vi "MainUI.vi"() -> ()   [LabVIEW 2012]
uses:
  Status.ctl
  StimulCtrls.lvlib
  Cohort.lvclass
  Sequence.lvclass
  SubPanels/InputPadRef.vi
  UserControl/RefWorkingFile.vi
  <vilib>/Utility/miscctls.llb/LVStringsAndValuesArrayTypeDef_U8.ctl
  UserControl/LeftPanel.ctl
  CohortConfig.ctl
  UserControl/ElectdPanel.ctl
  UserControl/ElectdTerminal.ctl
  UserControl/Cohort_sm.ctl
  SEQPool/SEQPool.ctl
panel:
  out "error out":errorcluster
  out "Current Time":timestamp format="%<%X\n%x>T"
  out "Lead #":string
  out "Left Panel":T1 {"Electrode 16"."Magnitude" format="%4.2f"; "Electrode 15"."Magnitude" format="%4.2f"; "Electrode 14"."Magnitude" format="%4.2f"; "Electrode 13"."Magnitude" format="%4.2f"; "Electrode 12"."Magnitude" format="%4.2f"; "Electrode 11"."Magnitude" format="%4.2f"; "Electrode 10"."Magnitude" format="%4.2f"; "Electrode 9"."Magnitude" format="%4.2f"; "Electrode 8"."Magnitude" format="%4.2f"; "Electrode 7"."Magnitude" format="%4.2f"; "Electrode 6"."Magnitude" format="%4.2f"; "Electrode 5"."Magnitude" format="%4.2f"; "Electrode 4"."Magnitude" format="%4.2f"; "Electrode 3"."Magnitude" format="%4.2f"; "Electrode 2"."Magnitude" format="%4.2f"; "Electrode"."Magnitude" format="%4.2f"}
  out "Stimulator #":string
  out "Physician ID":string
  out "Patient ID":string
  in  "stop":bool
  out "System Status":string
  in  "Mode Tab":T4(tab)
  in  "Seqn Open":bool
  in  "SetCathode":bool
  in  "SetAnode":bool
  in  "SetHiZ":bool
  in  "Assign Ten":bool
  in  "Assign Five":bool
  in  "Assign One":bool
  in  "Electd Select None":bool
  in  "Electd Sel All":bool
  in  "Cohort Undo":bool
  in  "Seqn Check":bool
  in  "Select a Cohort to Edit":u8(ring) items=["Cohort 0"]
  in  "Cohort Clear":bool
  in  "Cohort Add":bool
  in  "Cohort Delete":bool
  in  "Sequence Operation Log Saved to":path=path "C:/Users/zhengzhang/Documents/FRI_zz/TUI Project/Data/Cohorts.txt"
  in  "Seqn New":bool
  in  "Seqn Save as":bool
  out "Sequence Waveform Preview":dbl[](graph)
  in  "Cohort Panel":T5={"Frequency [Hz]"=55.0, "Pulse Width [ms]"=450.0, "Basic Unit"={"Electrode"={"Group #"="", "T #"=0, "Magnitude"=0.0, "check"=FALSE}, "Electrode 2"={"Group #"="", "T #"=0, "Magnitude"=0.0, "check"=FALSE}, "Electrode 3"={"Group #"="", "T #"=0, "Magnitude"=0.0, "check"=FALSE}, "Electrode 4"={"Group #"="", "T #"=0, "Magnitude"=0.0, "check"=FALSE}, "Electrode 5"={"Group #"="", "T #"=0, "Magnitude"=0.0, "check"=FALSE}, "Electrode 6"={"Group #"="", "T #"=0, "Magnitude"=0.0, "check"=FALSE}, "Electrode 7"={"Group #"="", "T #"=0, "Magnitude"=0.0, "check"=FALSE}, "Electrode 8"={"Group #"="", "T #"=0, "Magnitude"=0.0, "check"=FALSE}, "Electrode 9"={"Group #"="", "T #"=0, "Magnitude"=0.0, "check"=FALSE}, "Electrode 10"={"Group #"="", "T #"=0, "Magnitude"=0.0, "check"=FALSE}, "Electrode 11"={"Group #"="", "T #"=0, "Magnitude"=0.0, "check"=FALSE}, "Electrode 12"={"Group #"="", "T #"=0, "Magnitude"=0.0, "check"=FALSE}, "Electrode 13"={"Group #"="", "T #"=0, "Magnitude"=0.0, "check"=FALSE}, "Electrode 14"={"Group #"="", "T #"=0, "Magnitude"=0.0, "check"=FALSE}, "Electrode 15"={"Group #"="", "T #"=0, "Magnitude"=0.0, "check"=FALSE}, "Electrode 16"={"Group #"="", "T #"=0, "Magnitude"=0.0, "check"=FALSE}}, "Tag"=""} {"Pulse Width [ms]" format="%#.2f"; "Basic Unit"."Electrode 16"."Magnitude" format="%4.2f"; "Basic Unit"."Electrode 15"."Magnitude" format="%4.2f"; "Basic Unit"."Electrode 14"."Magnitude" format="%4.2f"; "Basic Unit"."Electrode 13"."Magnitude" format="%4.2f"; "Basic Unit"."Electrode 12"."Magnitude" format="%4.2f"; "Basic Unit"."Electrode 11"."Magnitude" format="%4.2f"; "Basic Unit"."Electrode 10"."Magnitude" format="%4.2f"; "Basic Unit"."Electrode 9"."Magnitude" format="%4.2f"; "Basic Unit"."Electrode 8"."Magnitude" format="%4.2f"; "Basic Unit"."Electrode 7"."Magnitude" format="%4.2f"; "Basic Unit"."Electrode 6"."Magnitude" format="%4.2f"; "Basic Unit"."Electrode 5"."Magnitude" format="%4.2f"; "Basic Unit"."Electrode 4"."Magnitude" format="%4.2f"; "Basic Unit"."Electrode 3"."Magnitude" format="%4.2f"; "Basic Unit"."Electrode 2"."Magnitude" format="%4.2f"; "Basic Unit"."Electrode"."Magnitude" format="%4.2f"}
  in  "Seqn Save":bool
  in  "Sequence List":i32(listbox)
  in  "PRG Preview":bool
  in  "PRG Setting":bool
  out "Pool":T6
  in  "Remove from Program":bool
  in  "Add to Program":bool
  in  "Prog Save as":bool
  in  "Pool Edit Seqn":bool
  in  "Pool Remove":bool
  in  "Pool Add":bool
  in  "Prog New":bool
  in  "Prog Save":bool
  in  "Prog Open":bool
  in  "Cycling Mode":bool=TRUE
  in  "Emergency Stop":bool
  out "Stimulation On":bool=TRUE
  in  "Battery (%)":dbl(slide)=62.51604621309371 scale=0.0..100.0
  in  "Signal Strength":dbl(slide)=79.58921694480102 scale=0.0..100.0
  out "Elapsed Time (min.)":dbl=30.0
  out "Experiment Duration (min.)":dbl=60.0
  out "Available ASIC Unit":dbl=2.0
  out "Available Memory":string="2 MB"
  out "ASIC Unit 1 On":bool=TRUE
  out "ASIC Unit 3 On":bool
  out "ASIC Unit 5 On":bool
  out "ASIC Unit 2 On":bool=TRUE
  out "ASIC Unit 4 On":bool
  out "ASIC Unit 6 On":bool
  out "Current Protocol":string="protocol 1"
  out "Current Program":string="program 1"
  out "Current Cycle":string="cycle 3"
  # "Experiment Profile"
  # "V 0.4 (Updated 6/26/2015)"
  # "Sequence Operation"
  # "Cohort Operation"
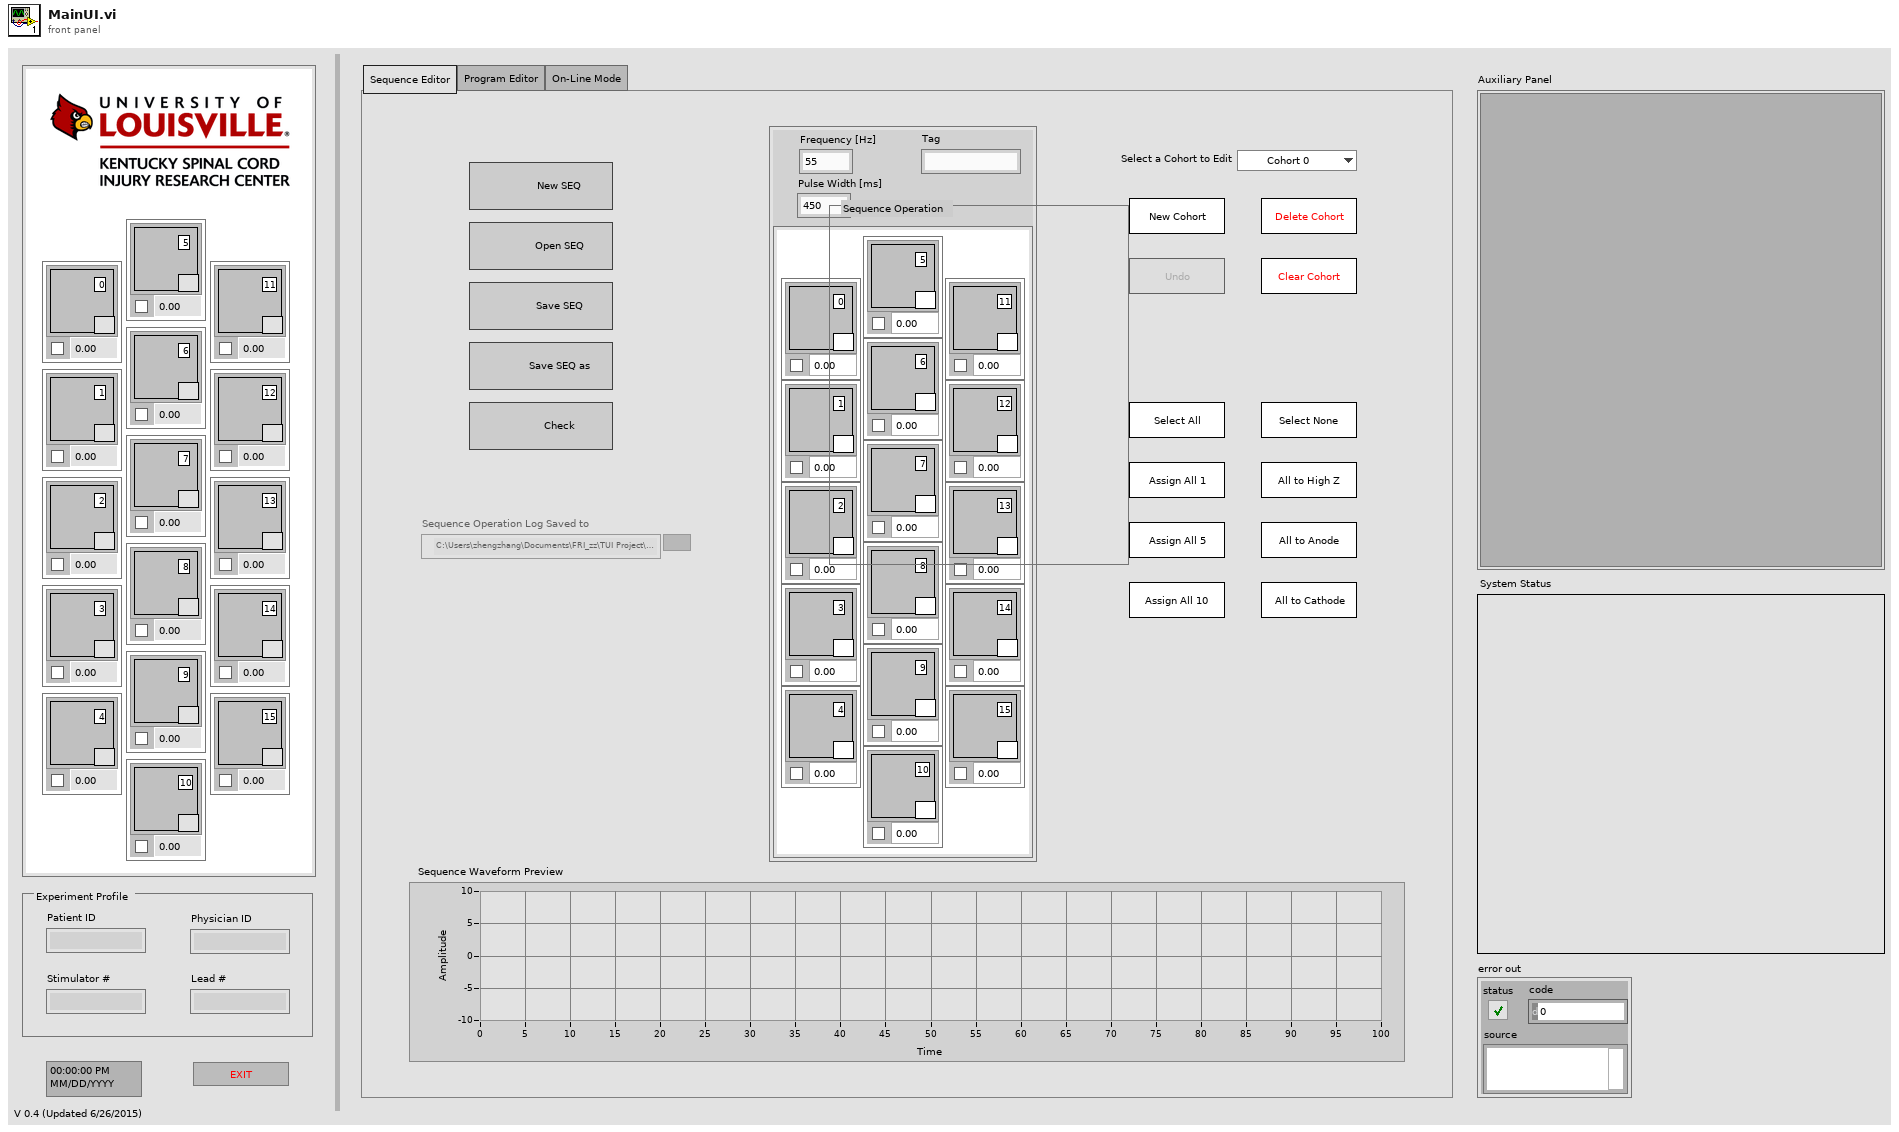
[diagram p1: front panel]
types:
  T1 = typedef "StimulCtrls.lvlib/LeftPanel.ctl" = cluster{"Electrode":T2, "Electrode 2":T2, "Electrode 3":T2, "Electrode 4":T2, "Electrode 5":T2, "Electrode 6":T2, "Electrode 7":T2, "Electrode 8":T2, "Electrode 9":T2, "Electrode 10":T2, "Electrode 11":T2, "Electrode 12":T2, "Electrode 13":T2, "Electrode 14":T2, "Electrode 15":T2, "Electrode 16":T2}
  T2 = typedef "StimulCtrls.lvlib/ElectdPanel.ctl" = cluster{"Group #":string, "T #":T3, "Magnitude":sgl, "check":bool}
  T3 = typedef "StimulCtrls.lvlib/ElectdTerminal.ctl" = u8
  T4 = enum32{"Sequence Editor", "Program Editor", "On-Line Mode"}
  T5 = typedef "StimulCtrls.lvlib/CohortConfig.ctl" = cluster{"Frequency [Hz]":sgl, "Pulse Width [ms]":sgl, "Basic Unit":T1, "Tag":string}
  T6 = typedef "StimulCtrls.lvlib/SEQPool.ctl" = cluster{"Seed 0":T7, "Seed 1":T7, "Seed 2":T7, "Seed 3":T7, "Seed 4":T7, "Seed 5":T7}
  T7 = typedef "StimulCtrls.lvlib/Cohort_sm.ctl" = cluster{"Ring 0":cluster{"T 0":T3}, "Ring 1":cluster{"T 0":T3}, "Ring 2":cluster{"T 0":T3}, "Ring 3":cluster{"T 0":T3}, "Ring 4":cluster{"T 0":T3}, "Ring 5":cluster{"T 0":T3}, "Ring 6":cluster{"T 0":T3}, "Ring 7":cluster{"T 0":T3}, "Ring 8":cluster{"T 0":T3}, "Ring 9":cluster{"T 0":T3}, "Ring 10":cluster{"T 0":T3}, "Ring 11":cluster{"T 0":T3}, "Ring 12":cluster{"T 0":T3}, "Ring 13":cluster{"T 0":T3}, "Ring 14":cluster{"T 0":T3}, "Ring 15":cluster{"T 0":T3}}
  T8 = typedef "StimulCtrls.lvlib/Status.ctl" = enum16{"SequenceOpen", "CohortShow", "Wait", "Stop", "UpdateLeftPanel", "SeqnSave", "CohortUpdate", "CohortAdd", "CohortClear", "CohortDel", "CohortBatch", "InputCall", "CohortCheck", "ProgQuit", "CohortQuickAmp", "CohortQuickState", "Initializing", "SeqnCheck", "PoolUpdate"}
  T9 = enum16{"open", "replace", "create", "open or create", "replace or create", "replace or create with confirmation"}
  T10 = enum16{"Add", "New", "Del", "Update", "Get", "Initial"}
  T11 = enum16{"Set", "Get", "Initial", "Change", "Saved"}
  T12 = enum8{"Enabled", "Disabled", "Disabled and Grayed Out"}
  T13 = typedef "LVStringsAndValuesArrayTypeDef_U8.ctl" = cluster{"String":string, "Value":u8}[]
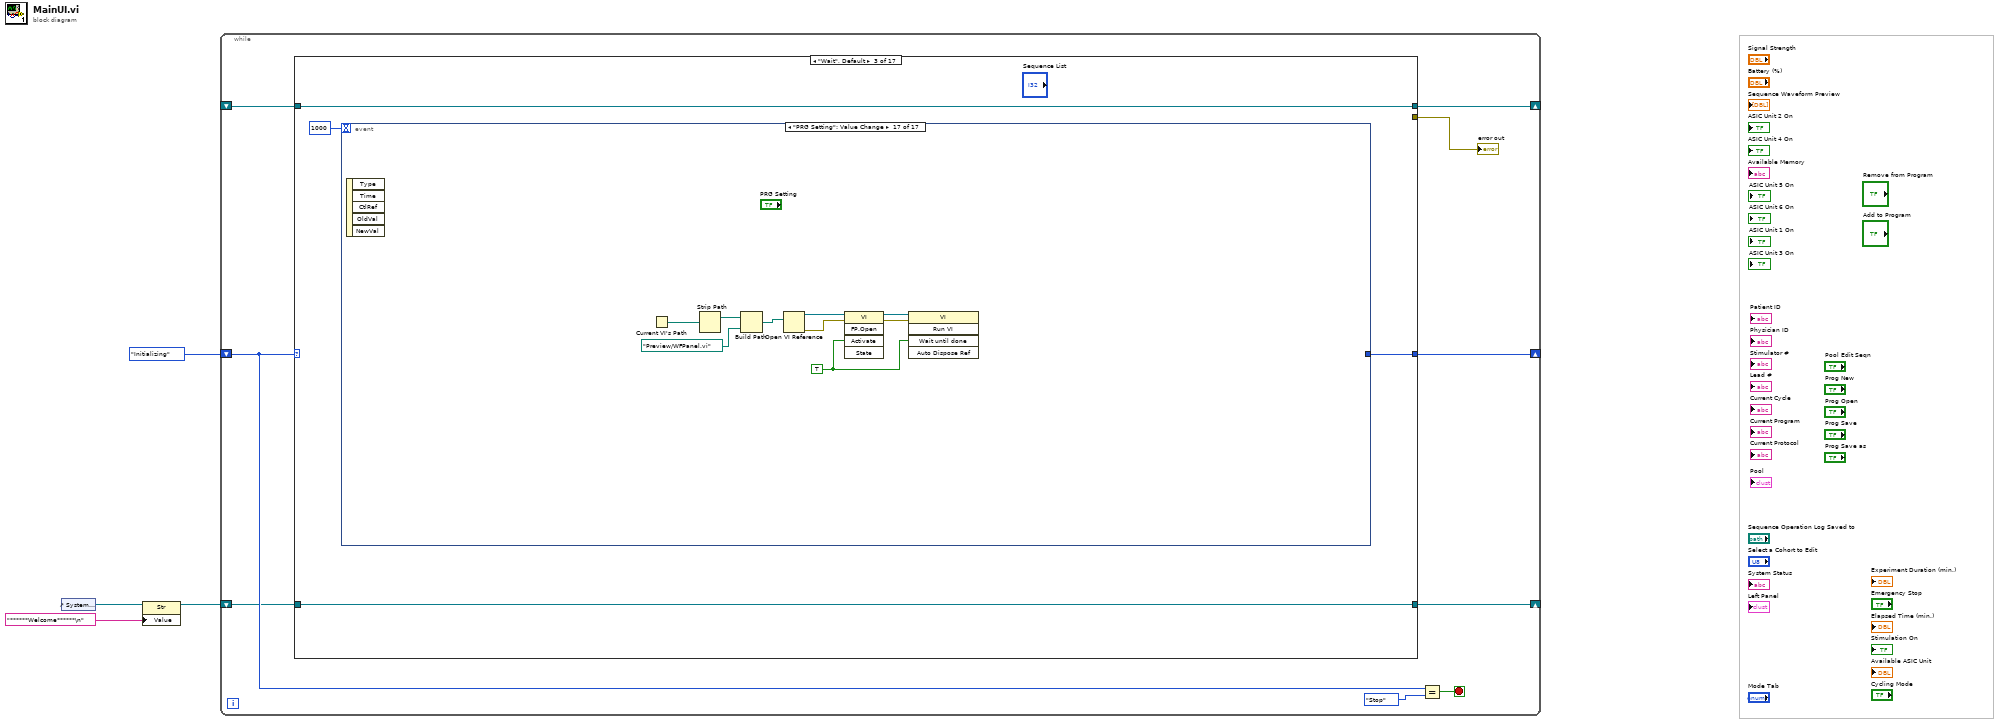
[diagram p0: block diagram]
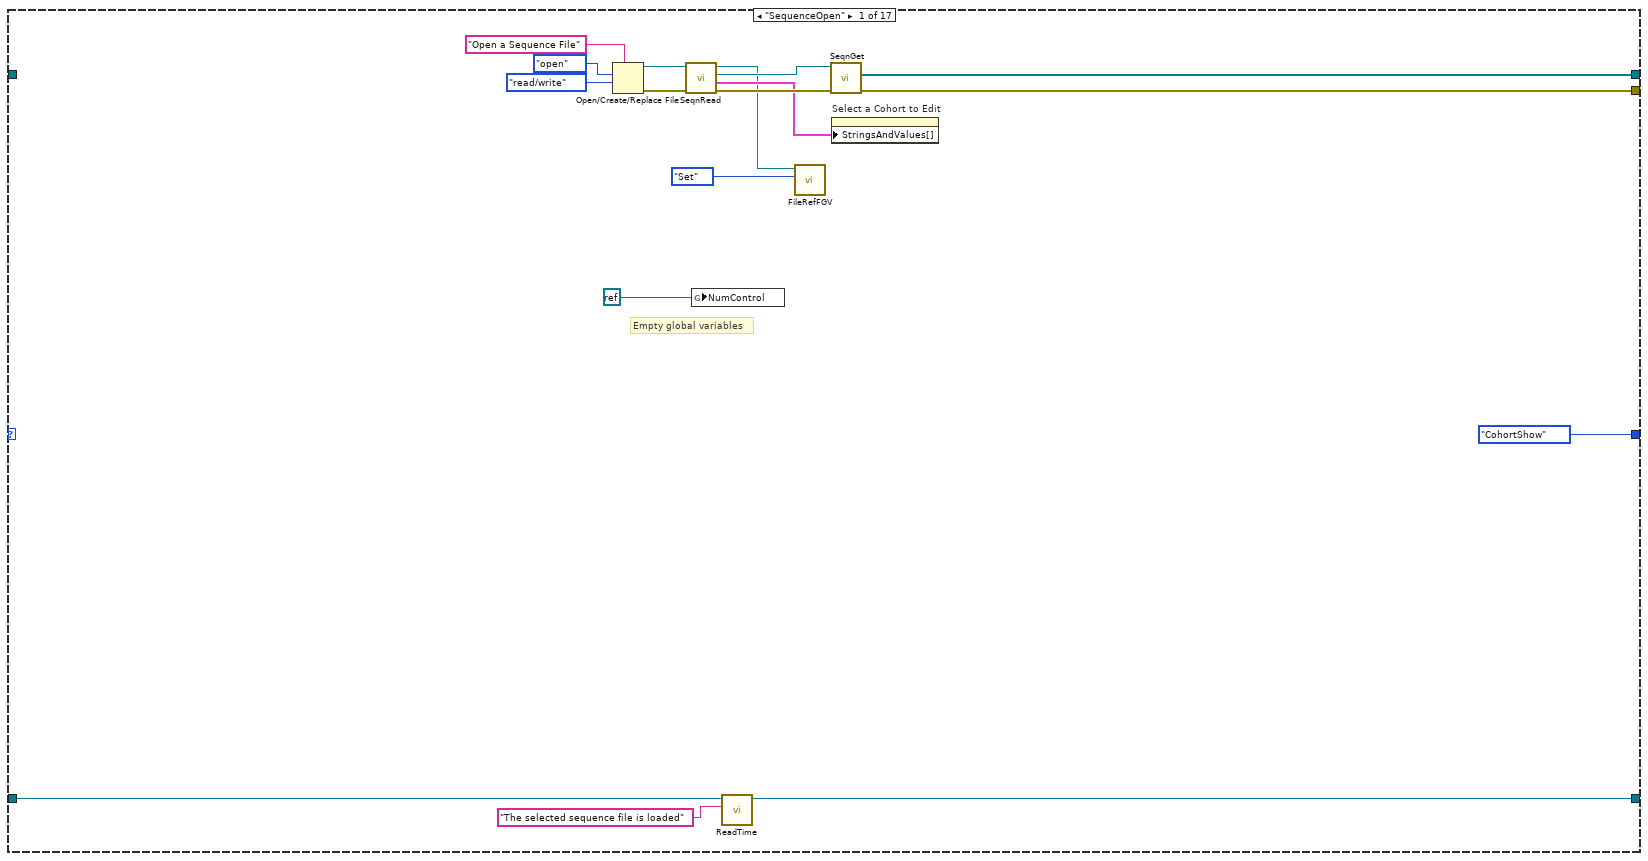
[diagram p2: hidden frame]
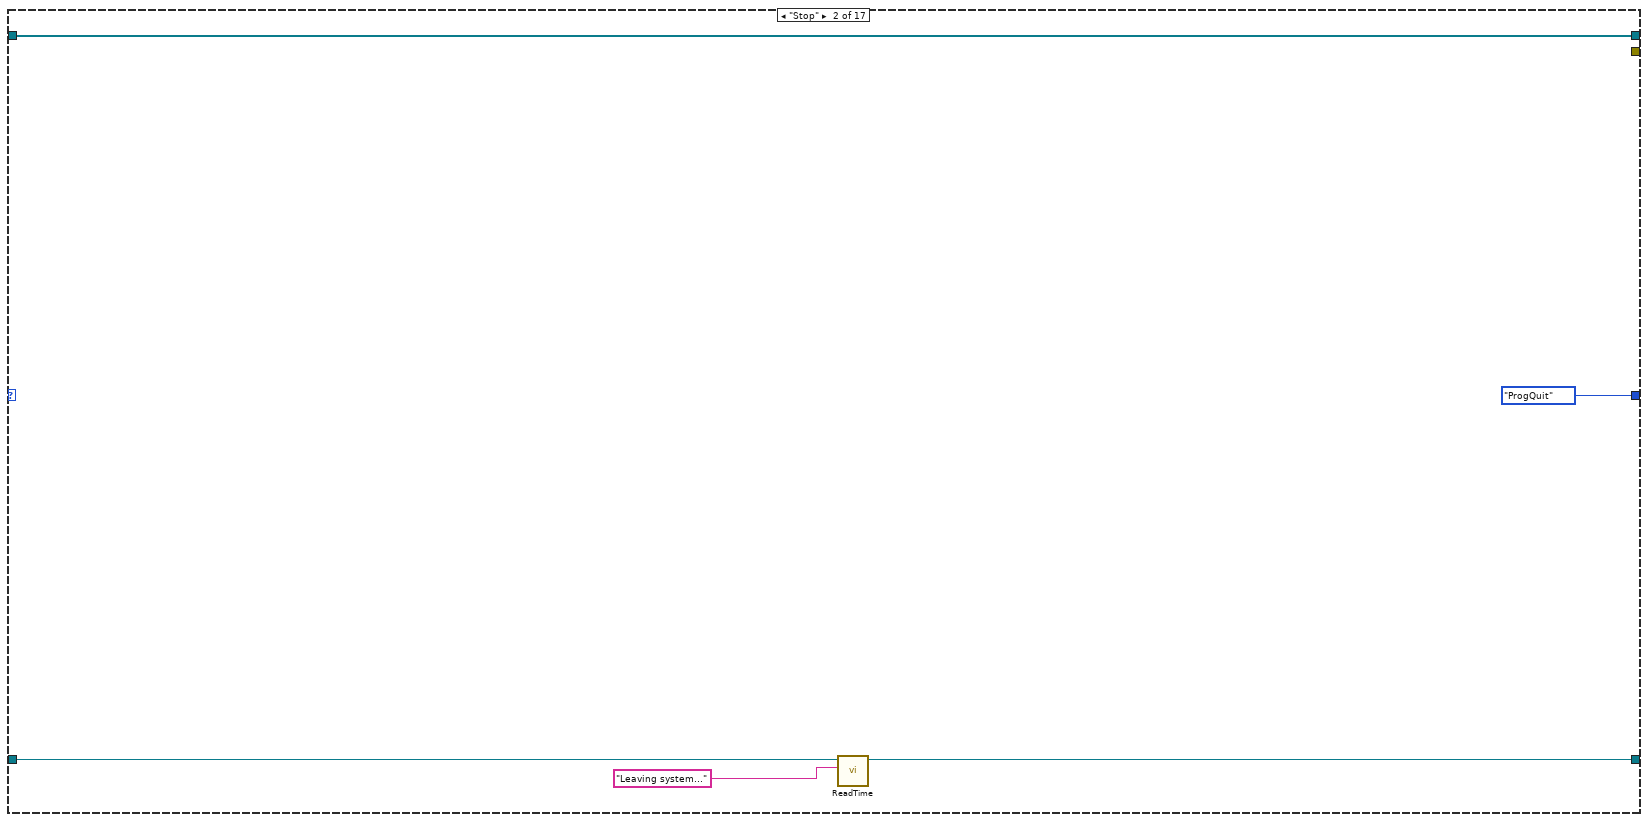
[diagram p3: hidden frame]
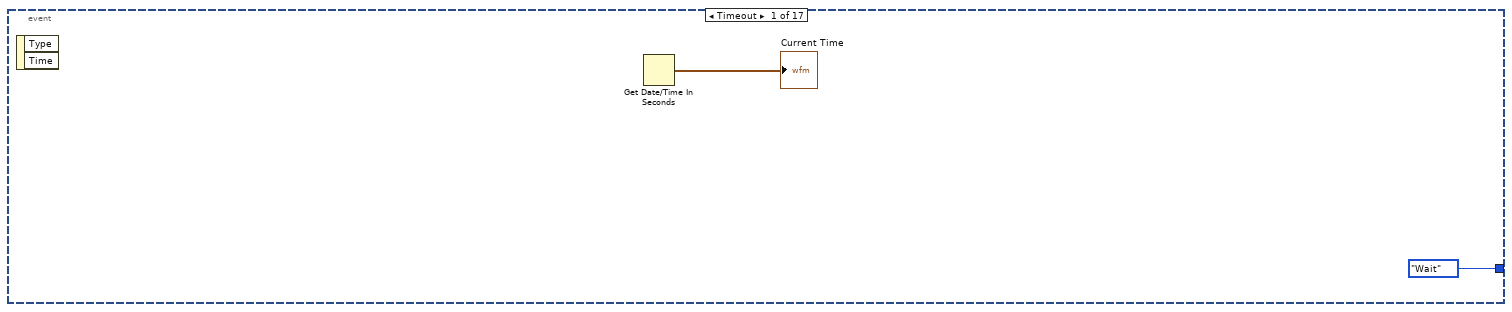
[diagram p4: hidden frame]
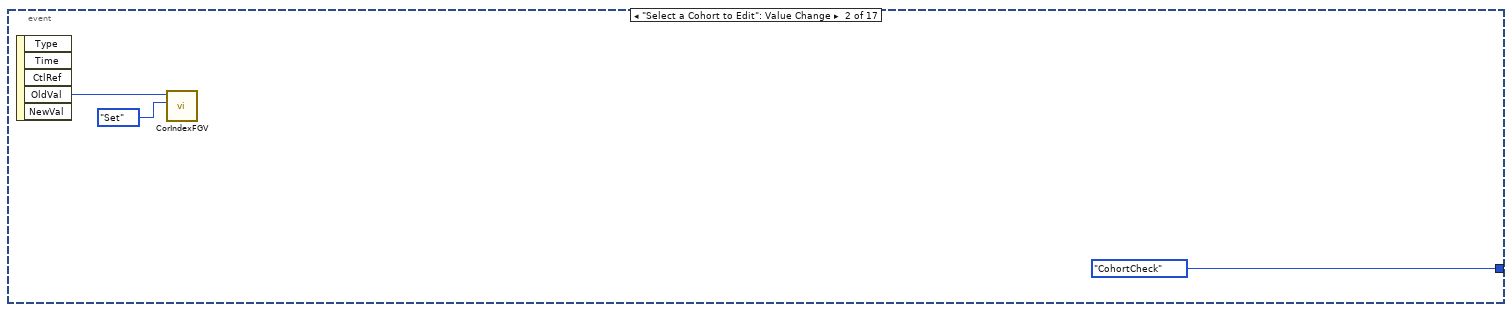
[diagram p5: hidden frame]
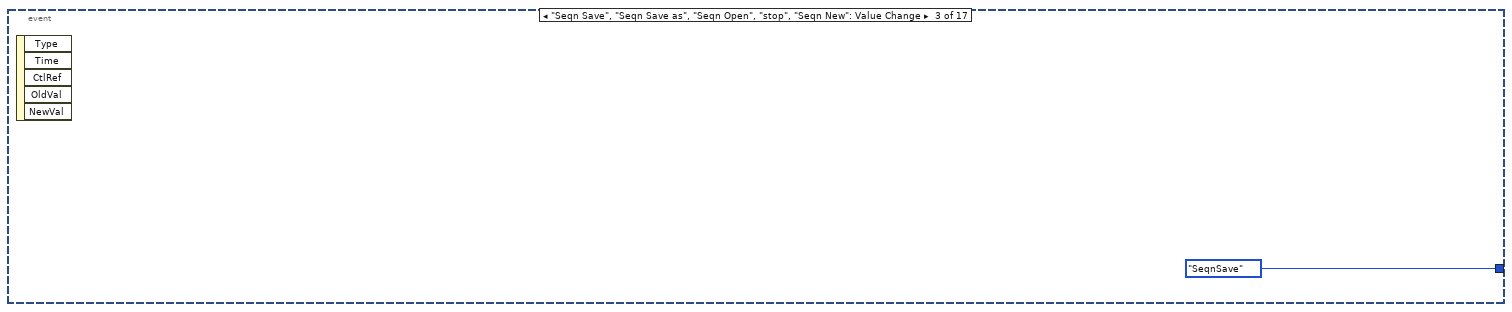
[diagram p6: hidden frame]
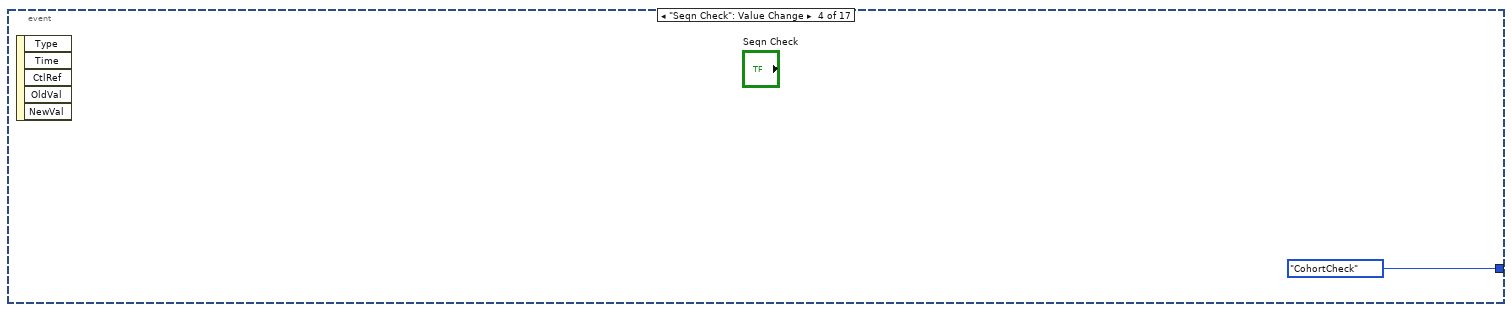
[diagram p7: hidden frame]
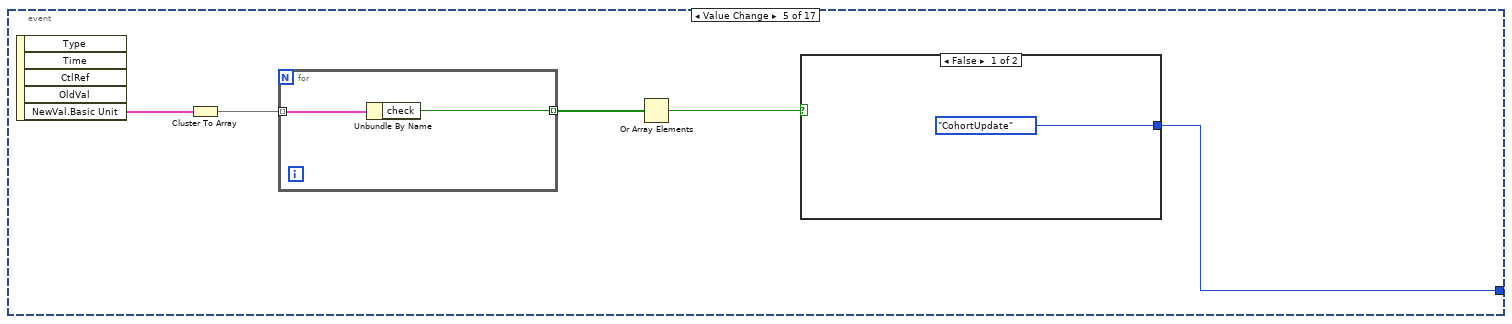
[diagram p8: hidden frame]
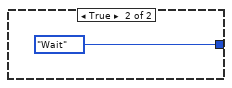
[diagram p9: hidden frame]
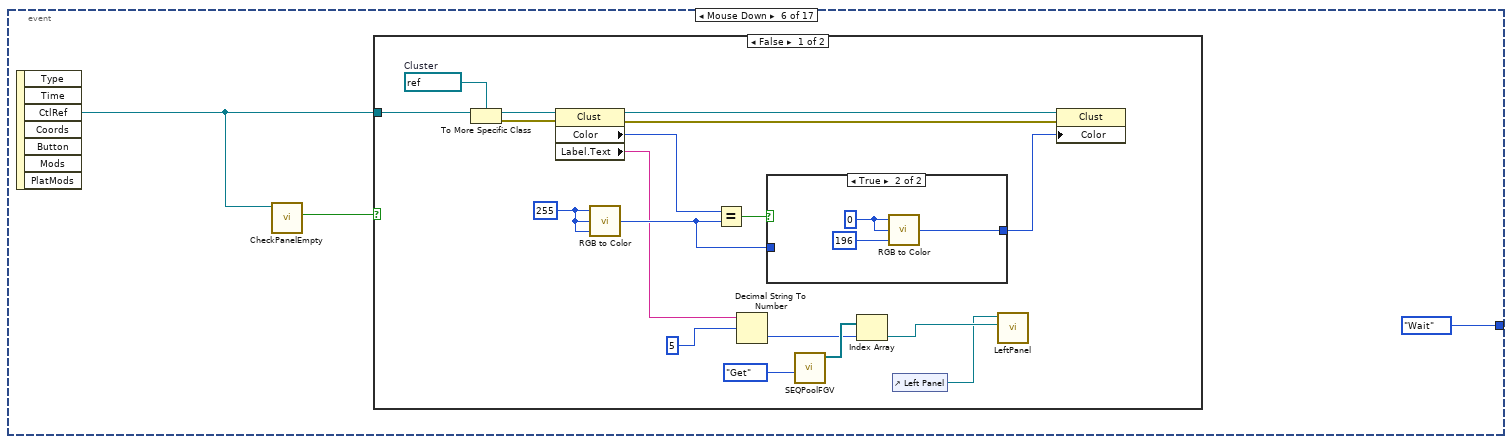
[diagram p10: hidden frame]
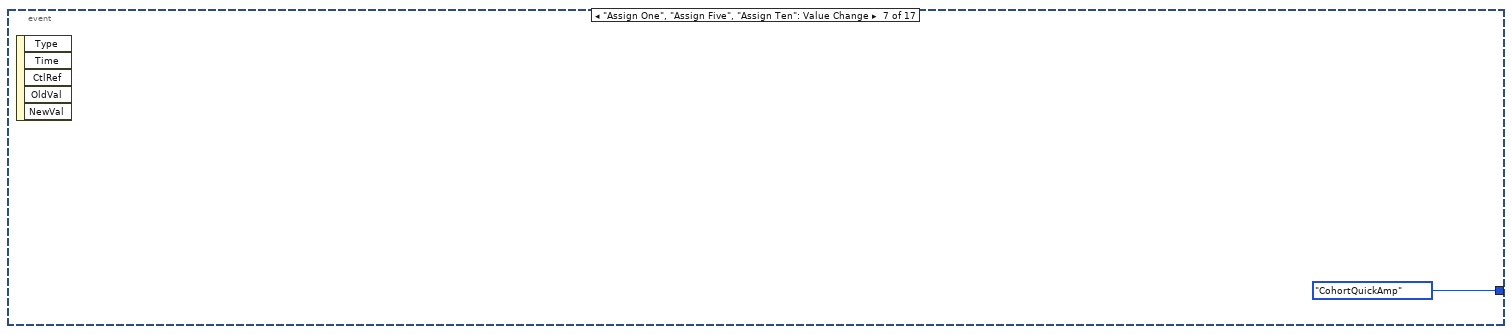
[diagram p13: hidden frame]
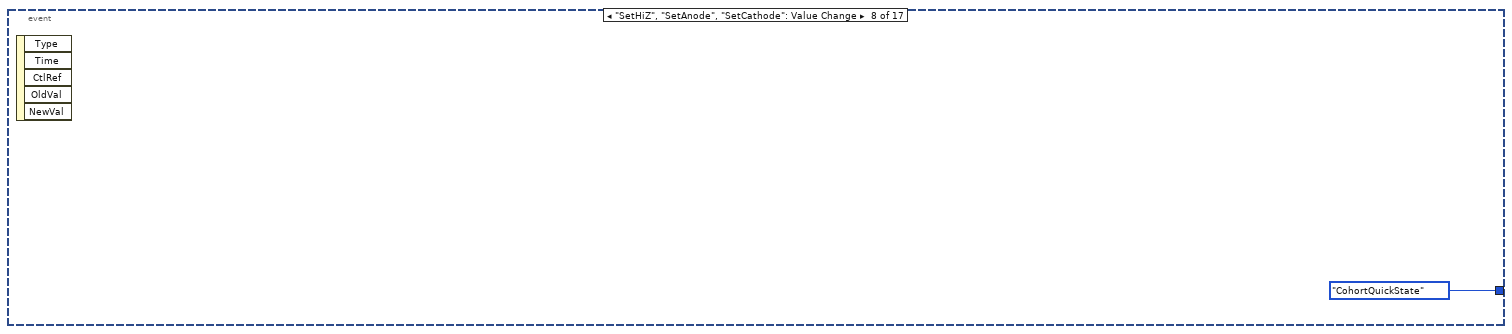
[diagram p14: hidden frame]
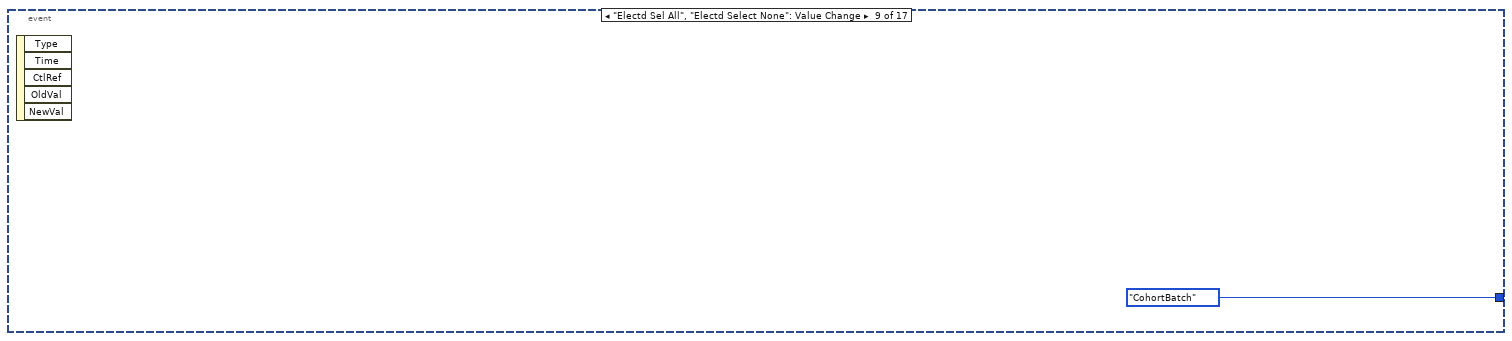
[diagram p15: hidden frame]
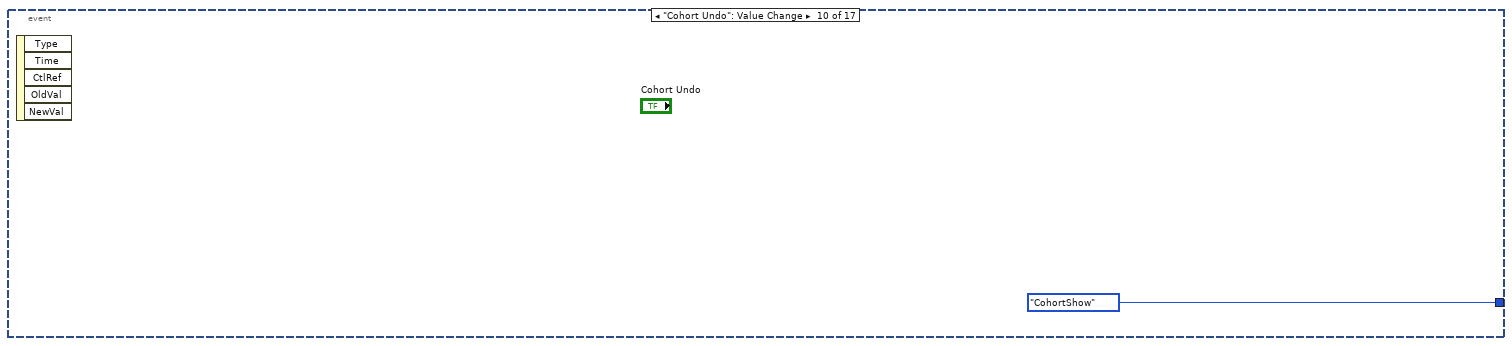
[diagram p16: hidden frame]
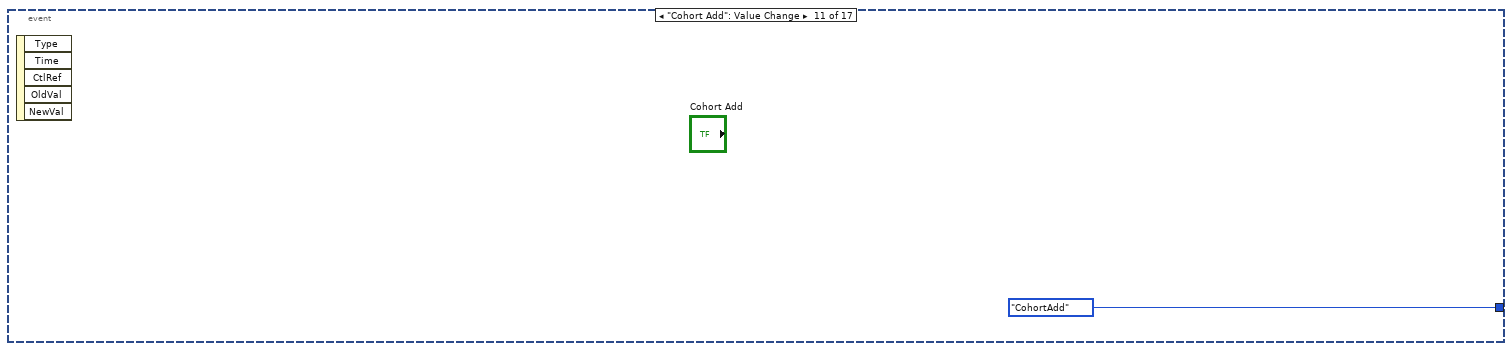
[diagram p17: hidden frame]
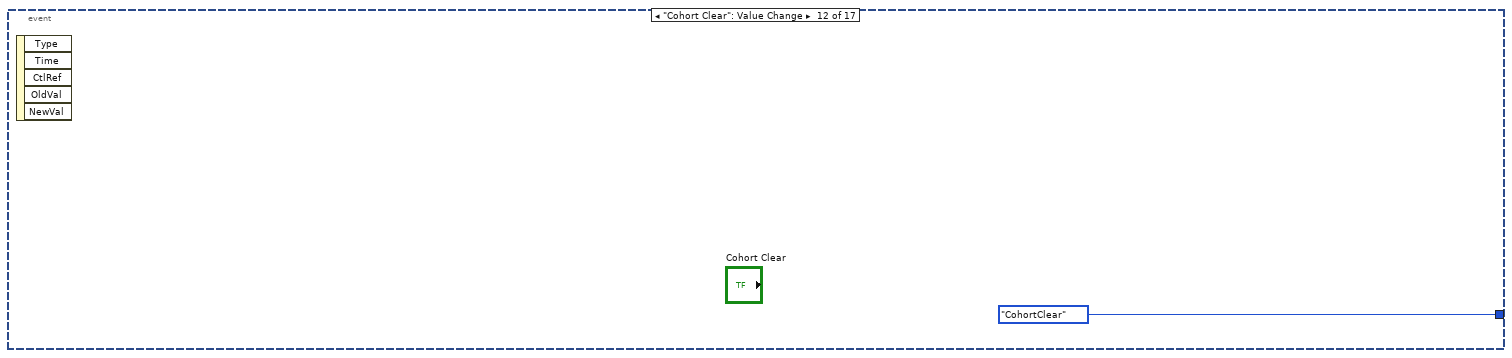
[diagram p18: hidden frame]
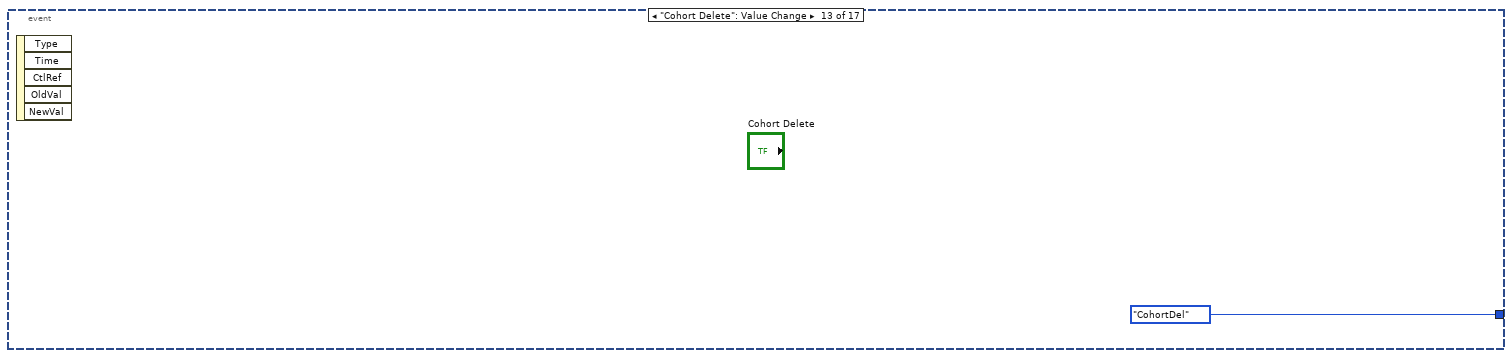
[diagram p19: hidden frame]
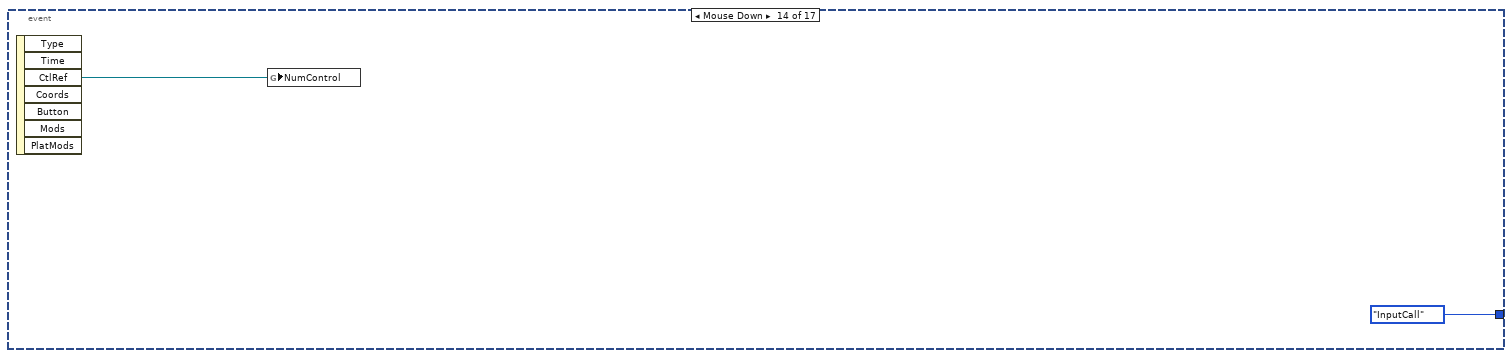
[diagram p20: hidden frame]
diagram:
  n1 = control-ref of="System Status"() -> (w1:refnum<vi>)
  n2 = property class="Str"(reference=w1, "Value"="******Welcome******\n" ("string")) -> (reference out=w3:refnum<vi>)  [unwired: 1 in, 1 out]
  n3 = while {
    shift-right: [w10] -> _
    shift-left: Status."Initializing" -> [w11]
    shift-right: [w9] -> _
    shift-left: _ -> [w8]
    shift-right: [w6] -> _
    shift-left: w3 -> [w7]
    stop <- w13 stop-if-true
    n4 = case shown="\"Wait\", Default" w11 {
      tunnel: [Status."CohortShow" Status."ProgQuit" w39 Status."Wait" w123 Status."CohortShow" Status."Wait" Status."CohortShow" Status."CohortShow" Status."UpdateLeftPanel" Status."CohortShow" Status."CohortUpdate" Status."CohortShow" Status."CohortUpdate" Status."CohortUpdate" Status."CohortShow" Status."UpdateLeftPanel"] -> w10
      tunnel: [w27 w34 w38 w114 w136 w184 w196 w233 w249 w256 w275 w307 w341 w349 w386 w418 w426] -> w9
      tunnel: w8 -> [_ w34 w38 w114 w136 w186 w196 w234 w251 w256 w276 w307 w341 w349 w386 _ w427]
      tunnel: w7 -> [w18 w32 w36 w113 w131 w174 w193 w231 w247 w254 w266 w290 w339 w348 w380 w415 w429]
      tunnel: [w17 w31 w36 w113 w130 w173 w193 w230 w246 w254 w265 w289 w339 w348 w380 w414 w429] -> w6
      tunnel: [w16 _ _ _ w122 w168 _ _ _ _ _ w281 _ _ _ _ w431] -> w5
      frame "SequenceOpen" {
        # "Empty global variables"
        n5 = Open/Create/Replace File(prompt="Open a Sequence File" ("prompt (Open existing file)"), operation (0:open)=T9."open", access (0:read/write)=enum16{"read/write", "read-only", "write-only"}."read/write") -> (refnum out=w25:refnum<file>, error out=w24:errorcluster)  [unwired: 3 in, 1 out]
        n6 = call "SeqnRead.vi"("error in (no error)"=w24, "File in Refnum"=w25) -> ("error out"=w28:errorcluster, "Cohort List"=w26:cluster{string, i32}[], "SEQ out"=w29:refnum<class "Sequence.lvclass">, "File out Refnum"=w14:refnum<file>)  [unwired: 6 in]
        n7 = global write "InputPadRef.vi" "NumControl"(refnum<k0> refnum) -> ()
        n8 = call "ReadTime.vi"("Input"="The selected sequence file is loaded", "Status in"=w18) -> ("Status out"=w17:refnum<vi>)  [unwired: 7 in]
        n9 = call "FileRefFGV.vi"("Action"=enum16{"Set", "Get", "Initial", "Change"}."Set", "File in"=w14) -> ()  [unwired: 8 in, 2 out]
        n10 = call-dynamic "SeqnGet.vi"("error in (no error)"=w28, "Sequence in"=w29) -> ("error out"=w16:errorcluster, "Cohorts"=w27:refnum<class "Cohort.lvclass">[])  [unwired: 7 in, 1 out]
        n11 = property on="Select a Cohort to Edit" class="Ring (strict)"("StringsAndValues[]"=w26) -> ()  [unwired: 2 in, 2 out]
      }
      frame "Stop" {
        n12 = call "ReadTime.vi"("Input"="Leaving system...", "Status in"=w32) -> ("Status out"=w31:refnum<vi>)  [unwired: 7 in]
      }
      frame "Wait", Default {
        n13 = event shown="[16] \"PRG Setting\": Value Change" {
          selector: _ -> [_ _ _ _ _ _ _ _ _ _ _ _ _ _ _ _ _]
          dyn-events: _ -> [_ _ _ _ _ _ _ _ _ _ _ _ _ _ _ _ _]
          timeout: 1000 -> [_ _ _ _ _ _ _ _ _ _ _ _ _ _ _ _ _]
          tunnel: [Status."Wait" Status."CohortCheck" Status."SeqnSave" Status."CohortCheck" w47 Status."Wait" Status."CohortQuickAmp" Status."CohortQuickState" Status."CohortBatch" Status."CohortShow" Status."CohortAdd" Status."CohortClear" Status."CohortDel" Status."InputCall" Status."PoolUpdate" Status."Wait" _] -> w39
          event Timeout {
            n14 = event-data() -> ()  [unwired: 1 in, 2 out]
            n15 = Get Date/Time In Seconds() -> (seconds since 1Jan1904=→"Current Time":timestamp)
          }
          event "Select a Cohort to Edit": Value Change {
            n16 = event-data() -> ("OldVal"=w43:u8)  [unwired: 1 in, 4 out]
            n17 = call "CorIndexFGV.vi"("Action"=enum16{"Set", "Get"}."Set", "Cohort Index"=w43) -> ()  [unwired: 9 in, 1 out]
          }
          event "Seqn Save", "Seqn Save as", "Seqn Open", "stop", "Seqn New": Value Change {
            n18 = event-data() -> ()  [unwired: 1 in, 5 out]
          }
          event "Seqn Check": Value Change {
            n19 = event-data() -> ()  [unwired: 1 in, 5 out]
          }
          event Value Change {
            n20 = event-data() -> ("NewVal.Basic Unit"=w51:T1)  [unwired: 1 in, 4 out]
            n21 = Cluster To Array(cluster=w51) -> (array=w50:T2[])
            n22 = for {
              tunnel: w50 -> [w55] mode=indexing
              tunnel: [w54] -> w49 mode=indexing
              n23 = Unbundle By Name(w55) -> ("check"=w54:bool)
            }
            n24 = Or Array Elements(Boolean array=w49) -> (logical OR=w48:bool)
            n25 = case shown="False" w48 {
              tunnel: [Status."CohortUpdate" Status."Wait"] -> w47
              frame False {
              }
              frame True {
              }
            }
          }
          event Mouse Down {
            n26 = event-data() -> ("CtlRef"=w57:refnum<vi>)  [unwired: 1 in, 6 out]
            n27 = call "CheckPanelEmpty.vi"("Panel in"=w57) -> ("Empty?"=w56:bool)  [unwired: 10 in]
            n28 = case shown="False" w56 {
              tunnel: w57 -> [w66 _]
              frame False {
                w73 = u8 255 ("R")
                w74 = refnum<vi> refnum  # Cluster
                n29 = To More Specific Class(target class=w74, reference=w66) -> (specific class reference=w76:refnum<vi>, error out=w75:errorcluster)  [unwired: 1 in]
                n30 = property class="Clust"(reference=w76, error in=w75) -> (reference out=w70:refnum<vi>, error out=w69:errorcluster, "Color"=w72:u32, "Label.Text"=w60:string)
                n31 = call <vilib>:"RGB to Color.vi"("B"=w73, "G"=w73, "R"=w73) -> ("Color"=w68:u32)
                n32 = Equal?(x=w72, y=w68) -> (x = y?=w71:bool)
                n33 = Decimal String To Number(string=w60, offset=5 ("offset (0)")) -> (number=w63:i32)  [unwired: 1 in, 1 out]
                n34 = case shown="True" w71 {
                  tunnel: w68 -> [w77 _]
                  tunnel: [w77 w78] -> w67
                  frame False {
                  }
                  frame True {
                    w80 = u8 0 ("R")
                    n35 = call <vilib>:"RGB to Color.vi"("B"=u8 196, "G"=w80, "R"=w80) -> ("Color"=w78:u32)
                  }
                }
                n36 = call "SEQPoolFGV.vi"("Action"=T10."Get") -> ("SEQ out"=w64:refnum<class "Sequence.lvclass">[])  [unwired: 10 in]
                n37 = Index Array(array=w64, index=w63) -> (element=w62:refnum<class "Sequence.lvclass">)
                n38 = control-ref of="Left Panel"() -> (w61:refnum<vi>)
                n39 = call "LeftPanel.vi"("Seqn in"=w62, "LP Refnum"=w61) -> ()  [unwired: 10 in]
                n40 = property class="Clust"(reference=w70, error in=w69, "Color"=w67) -> ()  [unwired: 2 out]
              }
              frame True {
              }
            }
          }
          event "Assign One", "Assign Five", "Assign Ten": Value Change {
            n41 = event-data() -> ()  [unwired: 1 in, 5 out]
          }
          event "SetHiZ", "SetAnode", "SetCathode": Value Change {
            n42 = event-data() -> ()  [unwired: 1 in, 5 out]
          }
          event "Electd Sel All", "Electd Select None": Value Change {
            n43 = event-data() -> ()  [unwired: 1 in, 5 out]
          }
          event "Cohort Undo": Value Change {
            n44 = event-data() -> ()  [unwired: 1 in, 5 out]
          }
          event "Cohort Add": Value Change {
            n45 = event-data() -> ()  [unwired: 1 in, 5 out]
          }
          event "Cohort Clear": Value Change {
            n46 = event-data() -> ()  [unwired: 1 in, 5 out]
          }
          event "Cohort Delete": Value Change {
            n47 = event-data() -> ()  [unwired: 1 in, 5 out]
          }
          event Mouse Down {
            n48 = event-data() -> ("CtlRef"=w88:refnum<vi>)  [unwired: 1 in, 6 out]
            n49 = global write "InputPadRef.vi" "NumControl"(w88) -> ()
          }
          event "Pool Add", "Pool Remove": Value Change {
            n50 = event-data() -> ()  [unwired: 1 in, 5 out]
          }
          event "PRG Preview": Value Change {
            n51 = event-data() -> ()  [unwired: 1 in, 5 out]
            n52 = Current VI's Path() -> (path=w99:path)
            n53 = Strip Path(path=w99) -> (stripped path=w100:path)  [unwired: 1 out]
            n54 = Build Path(base path=w100, name or relative path=path "Preview/WFPanel.vi" ("vi path")) -> (appended path=w98:path)
            n55 = Open VI Reference(vi path=w98) -> (vi reference=w96:refnum<vi>, error out=w95:errorcluster)  [unwired: 5 in]
            n56 = invoke class="VI" method="FP.Open"(reference=w96, error in=w95, "Activate"=TRUE ("Wait Until Done")) -> (reference out=w93:refnum<vi>, error out=w92:errorcluster)  [unwired: 2 in, 3 out]
            n57 = invoke class="VI" method="Run VI"(reference=w93, error in=w92, "Wait until done"=FALSE ("Wait Until Done")) -> ()  [unwired: 2 in, 5 out]
          }
          event "PRG Setting": Value Change {
            w102 = TRUE ("Wait Until Done")
            n58 = event-data() -> ()  [unwired: 1 in, 5 out]
            n59 = Current VI's Path() -> (path=w108:path)
            n60 = Strip Path(path=w108) -> (stripped path=w109:path)  [unwired: 1 out]
            n61 = Build Path(base path=w109, name or relative path=path "Preview/WFPanel.vi" ("vi path")) -> (appended path=w107:path)
            n62 = Open VI Reference(vi path=w107) -> (vi reference=w106:refnum<vi>, error out=w105:errorcluster)  [unwired: 5 in]
            n63 = invoke class="VI" method="FP.Open"(reference=w106, error in=w105, "Activate"=w102) -> (reference out=w104:refnum<vi>, error out=w103:errorcluster)  [unwired: 2 in, 3 out]
            n64 = invoke class="VI" method="Run VI"(reference=w104, error in=w103, "Wait until done"=w102) -> ()  [unwired: 2 in, 5 out]
          }
        }
      }
      frame "UpdateLeftPanel" {
        n65 = call "SeqnSet.vi"("Sequence"=w114) -> ("Sequence out"=w112:refnum<class "Sequence.lvclass">)  [unwired: 8 in, 1 out]
        n66 = control-ref of="Left Panel"() -> (w111:refnum<vi>)
        n67 = call "LeftPanel.vi"("Seqn in"=w112, "LP Refnum"=w111) -> ()  [unwired: 10 in]
      }
      frame "SeqnSave" {
        # "Save file?"
        # "File changed?"
        n68 = call "FileRefFGV.vi"("Action"=enum16{"Set", "Get", "Initial", "Change"}."Get") -> ("Changed?"=w120:bool)  [unwired: 9 in, 1 out]
        n69 = case shown="True" w120 {
          tunnel: [FALSE ("T button?") w140] -> w117
          frame False {
          }
          frame True {
            n70 = Two Button Dialog(message="Save current edit?", 1:"No" ("F button name (\"Cancel\")"), 2:"Yes" ("F button name (\"Cancel\")")) -> (T button?=w140:bool)
          }
        }
        n71 = Compound Arithmetic op=OR("Seqn Save as", w117, "Seqn Save") -> (w119:bool)
        n72 = case shown="True" w119 {
          tunnel: w136 -> [_ w150]
          tunnel: "Seqn Save as" -> [_ w148]
          tunnel: [errorcluster {"status"=FALSE, "code"=0, "source"=""} ("error out") w144] -> w122
          frame False {
          }
          frame True {
            n73 = case shown="False" w148 {
              tunnel: [w152 w158] -> w149
              tunnel: [w151 w157] -> w147
              frame True {
                n74 = Open/Create/Replace File(prompt="Create a New Cohort File", operation (0:open)=T9."replace or create") -> (refnum out=w152:refnum<file>, error out=w151:errorcluster)  [unwired: 4 in, 1 out]
                n75 = global write "RefWorkingFile.vi" "Working File Refnum"(w152) -> ()
              }
              frame False {
                n76 = call "FileRefFGV.vi"("Action"=enum16{"Set", "Get", "Initial", "Change"}."Get") -> ("File out"=w155:refnum<file>)  [unwired: 9 in, 1 out]
                n77 = Not Equal?(x=w155, y=refnum<k0> refnum) -> (x != y?=w159:bool)
                n78 = case shown="False" w159 {
                  tunnel: w155 -> [_ w166]
                  tunnel: [w162 w166] -> w158
                  tunnel: [w161 errorcluster {"status"=FALSE, "code"=0, "source"=""} ("error constant")] -> w157
                  frame False {
                    # "If file is no opened"
                    n79 = Open/Create/Replace File(prompt="Create a New Cohort File", operation (0:open)=T9."replace or create") -> (refnum out=w162:refnum<file>, error out=w161:errorcluster)  [unwired: 4 in, 1 out]
                    n80 = global write "RefWorkingFile.vi" "Working File Refnum"(w162) -> ()
                  }
                  frame True {
                  }
                }
              }
            }
            n81 = call "SeqnSet.vi"("Sequence"=w150, "error in (no error)"=w147) -> ("Sequence out"=w146:refnum<class "Sequence.lvclass">, "error out"=w145:errorcluster)  [unwired: 7 in]
            n82 = call "SeqnWrite.vi"("error in (no error)"=w145, "Seqn in"=w146, "File in Refnum"=w149) -> ("error out"=w144:errorcluster)  [unwired: 8 in]
            n83 = call "FileRefFGV.vi"("Action"=T11."Saved") -> ()  [unwired: 9 in, 2 out]
          }
        }
        n84 = call "ReadTime.vi"("Input"="The current sequence is saved", "Status in"=w131) -> ("Status out"=w130:refnum<vi>)  [unwired: 7 in]
        n85 = Select(t=Status."Initializing", s="Seqn New", f=Status."Wait") -> (s? t:f=w128:T8)
        n86 = Select(t=Status."SequenceOpen", s="Seqn Open", f=w128) -> (s? t:f=w126:T8)
        n87 = Select(t=Status."Stop", s="stop", f=w126) -> (s? t:f=w123:T8)
      }
      frame "CohortAdd" {
        w188 = u8 1 ("Set Pulse Frequency")
        # "To create an automatic tag for the new cohort in the ring\nNew cohort will be appended to the sequence"
        # "Append the new cohort to the array"
        # "Initialize a new, empty cohort"
        n88 = control-ref of="Select a Cohort to Edit"() -> (w183:refnum<vi>)
        n89 = property class="Ring (strict)"(reference=w183) -> (reference out=w182:refnum<vi>, error out=w169:errorcluster, "StringsAndValues[]"=w177:T13, "NumItems"=w172:u32)  [unwired: 1 in]
        n90 = Initialize Array(-1, 16 ("dimension size")) -> (w189:i32[])
        n91 = Number To Decimal String(number=w172, width (-)=i16 2) -> (decimal integer string=w179:string)
        n92 = Concatenate Strings("Cohort", w179) -> (w170:string)
        n93 = call "CohortSet.vi"("Set COR Tag"=w170, "Set Electrodes"=w189, "Set Pulse Width"=w188, "Set Pulse Frequency"=w188) -> ("Cohort out"=w185:refnum<class "Cohort.lvclass">)  [unwired: 6 in, 1 out]
        n94 = Bundle(w170, "NumItems"=w172) -> (w176:cluster{string, "NumItems":u32})  [unwired: 1 in]
        n95 = call "CorIndexFGV.vi"("Action"=enum16{"Set", "Get"}."Set", "Cohort Index"=w172) -> ()  [unwired: 9 in, 1 out]
        n96 = call "FileRefFGV.vi"("Action"=enum16{"Set", "Get", "Initial", "Change"}."Change") -> ()  [unwired: 9 in, 2 out]
        n97 = Build Array (concatenate)(w177, w176) -> (w178:cluster{"String":string, "NumItems":u32}[])
        n98 = call "ReadTime.vi"("Input"="A empty cohort is appended to the current sequence", "Status in"=w174) -> ("Status out"=w173:refnum<vi>)  [unwired: 7 in]
        n99 = Insert Into Array(array=w186, new element=w185) -> (w184:refnum<class "Cohort.lvclass">[])  [unwired: 1 in]
        n100 = property class="Ring (strict)"(reference=w182, error in=w169, "StringsAndValues[]"=w178) -> (error out=w168:errorcluster)  [unwired: 1 out]
      }
      frame "CohortBatch" {
        w199 = refnum<vi> refnum  # Cluster
        # "Electrode"
        n101 = control-ref of="Cohort Panel"() -> (w204:refnum<vi>)
        n102 = property class="Clust (strict)"(reference=w204) -> ("Controls[]"=w203:refnum<vi>[])  [unwired: 1 in, 2 out]
        n103 = Index Array(array=w203, index=2) -> (element=w201:refnum<vi>)
        n104 = To More Specific Class(target class=w199, reference=w201) -> (specific class reference=w200:refnum<vi>)  [unwired: 1 in, 1 out]
        n105 = property class="Clust"(reference=w200) -> ("Controls[]"=w198:refnum<vi>[])  [unwired: 1 in, 2 out]
        n106 = for {
          tunnel: w198 -> [w220] mode=indexing
          tunnel: "Electd Sel All" -> [w209]
          tunnel: "Electd Select None" -> [w205]
          w216 = refnum<vi> refnum  # Boolean
          w221 = refnum<vi> refnum  # Cluster
          # "Select All"
          # "Select None"
          # "Checkbox"
          n107 = To More Specific Class(target class=w221, reference=w220) -> (specific class reference=w219:refnum<vi>)  [unwired: 1 in, 1 out]
          n108 = property class="Clust"(reference=w219) -> ("Controls[]"=w217:refnum<vi>[])  [unwired: 1 in, 2 out]
          n109 = Index Array(array=w217, index=3) -> (element=w215:refnum<vi>)
          n110 = To More Specific Class(target class=w216, reference=w215) -> (specific class reference=w206:refnum<vi>)  [unwired: 1 in, 1 out]
          n111 = case shown="True" w205 {
            tunnel: w206 -> [_ w223]
            frame False {
            }
            frame True {
              n112 = property class="Bool"(reference=w223, "Value"=FALSE) -> ()  [unwired: 1 in, 2 out]
            }
          }
          n113 = property class="Bool"(reference=w206) -> (reference out=w208:refnum<vi>, "DisabledEnum"=w214:T12)  [unwired: 1 in, 1 out]
          n114 = Equal?(x=w214, y=T12."Enabled") -> (x = y?=w212:bool)
          n115 = Select(t=TRUE, s=w212, f=FALSE) -> (s? t:f=w207:bool)
          n116 = case shown="True" w209 {
            tunnel: w208 -> [_ w225]
            tunnel: w207 -> [_ w224]
            frame False {
            }
            frame True {
              n117 = property class="Bool"(reference=w225, "Value"=w224) -> ()  [unwired: 1 in, 2 out]
            }
          }
        }
        n118 = call "FileRefFGV.vi"("Action"=enum16{"Set", "Get", "Initial", "Change"}."Change") -> ()  [unwired: 9 in, 2 out]
      }
      frame "CohortClear" {
        w236 = u8 1 ("Set Pulse Frequency")
        n119 = Initialize Array(-1, 16 ("dimension size")) -> (w237:i32[])
        n120 = call "CohortSet.vi"("Set COR Tag"="", "Set Electrodes"=w237, "Set Pulse Width"=w236, "Set Pulse Frequency"=w236) -> ("Cohort out"=w235:refnum<class "Cohort.lvclass">)  [unwired: 6 in, 1 out]
        n121 = call "CorIndexFGV.vi"("Action"=enum16{"Set", "Get"}."Get") -> ("New Index"=w229:u8)  [unwired: 10 in]
        n122 = call "ReadTime.vi"("Input"="The current cohort is cleared", "Status in"=w231) -> ("Status out"=w230:refnum<vi>)  [unwired: 7 in]
        n123 = call "FileRefFGV.vi"("Action"=enum16{"Set", "Get", "Initial", "Change"}."Change") -> ()  [unwired: 9 in, 2 out]
        n124 = Replace Array Subset(array=w234, new element=w235, index=w229) -> (w233:refnum<class "Cohort.lvclass">[])
      }
      frame "CohortDel" {
        n125 = property on="Select a Cohort to Edit" class="Ring (strict)"() -> ("Strings []"=w244:string[])  [unwired: 2 in, 2 out]
        n126 = call "CorIndexFGV.vi"("Action"=enum16{"Set", "Get", "Del"}."Del") -> ("New Index"=w243:u8)  [unwired: 10 in]
        n127 = call "FileRefFGV.vi"("Action"=enum16{"Set", "Get", "Initial", "Change"}."Change") -> ()  [unwired: 9 in, 2 out]
        n128 = Delete From Array(array=w251, index=w243) -> (array with subset deleted=w249:refnum<class "Cohort.lvclass">[])  [unwired: 1 in, 1 out]
        n129 = Delete From Array(array=w244, index=w243) -> (array with subset deleted=w245:string[])  [unwired: 1 in, 1 out]
        n130 = call "ReadTime.vi"("Input"="The cohort is deleted", "Status in"=w247) -> ("Status out"=w246:refnum<vi>)  [unwired: 7 in]
        n131 = property on="Select a Cohort to Edit" class="Ring (strict)"("Strings []"=w245) -> ()  [unwired: 2 in, 2 out]
      }
      frame "CohortShow" {
        n132 = call "CorIndexFGV.vi"("Action"=enum16{"Set", "Get", "Del"}."Get") -> ("New Index"=w252:u8)  [unwired: 10 in]
        n133 = control-ref of="Cohort Panel"() -> (w255:refnum<vi>)
        n134 = call "CohortShowCohort.vi"("Group #"=w252, "Cohorts in"=w256, "Coh Panel in"=w255) -> ()  [unwired: 4 in, 3 out]
        n135 = property on="Select a Cohort to Edit" class="Ring (strict)"("Value"=w252) -> ()  [unwired: 2 in, 2 out]
      }
      frame "CohortUpdate" {
        n136 = Unbundle By Name("Cohort Panel") -> ("Frequency [Hz]"=w272:sgl, "Pulse Width [ms]"=w271:sgl, "Basic Unit"=w270:T1, "Tag"=w262:string)
        n137 = Cluster To Array(cluster=w270) -> (array=w269:T2[])
        n138 = for {
          tunnel: w269 -> [w279] mode=indexing
          tunnel: [w278] -> w274 mode=indexing
          n139 = call "RingToAmp.vi"("Electrode"=w279) -> ("Amplitude"=w278:sgl)  [unwired: 10 in]
        }
        n140 = call "ReadTime.vi"("Input"="The cohort is updated", "Status in"=w266) -> ("Status out"=w265:refnum<vi>)  [unwired: 7 in]
        n141 = property on="Select a Cohort to Edit" class="Ring (strict)"() -> (error out=w260:errorcluster, "Strings []"=w264:string[])  [unwired: 2 in, 1 out]
        n142 = call "FileRefFGV.vi"("Action"=enum16{"Set", "Get", "Initial", "Change"}."Change") -> ()  [unwired: 9 in, 2 out]
        n143 = call "CorIndexFGV.vi"("Action"=enum16{"Set", "Get", "Del"}."Get") -> ("New Index"=w259:u8)  [unwired: 10 in]
        n144 = call "CohortSet.vi"("Set COR Tag"=w262, "Set Electrodes"=w274, "Set Pulse Width"=w271, "Set Pulse Frequency"=w272) -> ("Cohort out"=w268:refnum<class "Cohort.lvclass">)  [unwired: 6 in, 1 out]
        n145 = Replace Array Subset(array=w264, new element=w262, index=w259) -> (w261:string[])
        n146 = Replace Array Subset(array=w276, new element=w268, index=w259) -> (w275:refnum<class "Cohort.lvclass">[])
        n147 = property on="Select a Cohort to Edit" class="Ring (strict)"(error in=w260, "Strings []"=w261) -> ()  [unwired: 1 in, 2 out]
      }
      frame "InputCall" {
        # "Update Data"
        # "Load Input Pad"
        n148 = global read "InputPadRef.vi" "NumControl"() -> (w287:refnum<vi>)
        n149 = Current VI's Path() -> (path=w295:path)
        n150 = Strip Path(path=w295) -> (stripped path=w296:path)  [unwired: 1 out]
        n151 = property class="Ctl"(reference=w287) -> (error out=w284:errorcluster, "Value"=w286:variant)  [unwired: 1 in, 1 out]
        n152 = vi-ref "InputPad.vi"() -> (w305:refnum<vi>)
        n153 = Build Path(base path=w296, name or relative path=path "SubPanels/inputpad.vi" ("vi path")) -> (appended path=w297:path)
        n154 = Open VI Reference(type specifier VI Refnum (for type only)=w305, vi path=w297, options=256) -> (vi reference=w293:refnum<vi>, error out=w288:errorcluster)  [unwired: 3 in]
        n155 = Variant To Data(error in=w284, type=sgl 0.0, Variant=w286) -> (data=w285:sgl)  [unwired: 1 out]
        n156 = call-by-ref "Start Asynchronous Call"(reference=w293, error in=w288, "Num in"=w285) -> (reference out=w294:refnum<vi>, error out=w292:errorcluster)  [unwired: 10 in, 1 out]
        n157 = property class="Ctl"(reference=w287) -> ("Label.Text"=w301:string)  [unwired: 1 in, 2 out]
        n158 = call-by-ref "Wait On Asynchronous Call"(reference=w294, error in=w292) -> (reference out=w302:refnum<vi>, error out=w303:errorcluster, "Num out"=w282:dbl)  [unwired: 11 in]
        n159 = case shown="Default" w301 {
          tunnel: w303 -> [w309 w316]
          tunnel: w302 -> [w312 w317]
          tunnel: w282 -> [w310 w313]
          tunnel: w287 -> [w311 w314]
          tunnel: [w312 w317] -> w300
          tunnel: [w308 w316] -> w299
          frame "Frequency [Hz]", "Pulse Width [ms]" {
            n160 = property class="Ctl"(reference=w311, error in=w309, "Value"=w310) -> (error out=w308:errorcluster)  [unwired: 1 out]
          }
          frame Default {
            n161 = property on="Basic Unit" class="Clust (strict)"() -> ("Controls[]"=w315:refnum<vi>[])  [unwired: 2 in, 2 out]
            n162 = for {
              tunnel: w313 -> [w332]
              tunnel: w314 -> [_]
              tunnel: w315 -> [w326] mode=indexing
              w331 = refnum<vi> refnum  # Cluster
              n163 = To More Specific Class(target class=w331, reference=w326) -> (specific class reference=w330:refnum<vi>, error out=w327:errorcluster)  [unwired: 1 in]
              n164 = property class="Clust"(reference=w330, error in=w327) -> (error out=w322:errorcluster, "Controls[]"=w329:refnum<vi>[])  [unwired: 1 out]
              n165 = Index Array(array=w329, index #1=3 ("index"), index #2=2 ("index")) -> (element #1=w323:refnum<vi>, element #2=w324:refnum<vi>)
              n166 = property class="Ctl"(reference=w323, error in=w322) -> (error out=w321:errorcluster, "Value"=w320:variant)  [unwired: 1 out]
              n167 = Variant To Data(error in=w321, type=TRUE, Variant=w320) -> (data=w319:bool)  [unwired: 1 out]
              n168 = case shown="True" w319 {
                tunnel: w332 -> [_ w333]
                tunnel: w324 -> [_ w336]
                frame False {
                }
                frame True {
                  w335 = refnum<vi> refnum  # Numeric
                  n169 = To More Specific Class(target class=w335, reference=w336) -> (specific class reference=w334:refnum<vi>)  [unwired: 1 in, 1 out]
                  n170 = property class="Num"(reference=w334, "Value"=w333) -> ()  [unwired: 1 in, 2 out]
                }
              }
            }
            n171 = property class="Ctl"(reference=w314, "Value"=w313) -> ()  [unwired: 1 in, 2 out]
          }
        }
        n172 = call "FileRefFGV.vi"("Action"=enum16{"Set", "Get", "Initial", "Change"}."Change") -> ()  [unwired: 9 in, 2 out]
        n173 = call "ReadTime.vi"("Input"="Input the value using right panel", "Status in"=w290) -> ("Status out"=w289:refnum<vi>)  [unwired: 7 in]
        n174 = Close Reference(reference=w300, error in (no error)=w299) -> (error out=w281:errorcluster)
      }
      frame "CohortCheck" {
        # "Check cohort configuration"
        n175 = call "CorIndexFGV.vi"("Action"=enum16{"Set", "Get", "Del"}."Get") -> ("New Index"=w337:u8)  [unwired: 10 in]
        n176 = Index Array(array=w341, index=w337) -> (element=w342:refnum<class "Cohort.lvclass">)
        n177 = call "CohortCheck.vi"("Cohort in"=w342) -> ("error out"=w343:errorcluster)  [unwired: 10 in]
        n178 = case shown="No Error" w343 {
          frame No Error {
            n179 = property on="Select a Cohort to Edit" class="Ring (strict)"() -> ("Value"=w344:u8)  [unwired: 2 in, 2 out]
            n180 = call "CorIndexFGV.vi"("Action"=enum16{"Set", "Get", "Del"}."Set", "Cohort Index"=w344) -> ()  [unwired: 9 in, 1 out]
          }
          frame Error {
            n181 = One Button Dialog(message="Cohort is not completed") -> ()  [unwired: 1 in, 1 out]
          }
        }
      }
      frame "CohortQuickAmp" {
        n182 = property on="Basic Unit" class="Clust (strict)"() -> ("Controls[]"=w364:refnum<vi>[])  [unwired: 2 in, 2 out]
        n183 = Select(t=1, s="Assign One", f=0) -> (s? t:f=w353:i32)
        n184 = Select(t=5, s="Assign Five", f=0) -> (s? t:f=w352:i32)
        n185 = Select(t=10, s="Assign Ten", f=0) -> (s? t:f=w351:i32)
        n186 = Compound Arithmetic op=ADD(w353, w352, w351) -> (w350:i32)
        n187 = for {
          tunnel: w364 -> [w376] mode=indexing
          tunnel: w350 -> [w365]
          w375 = refnum<vi> refnum  # Cluster
          n188 = To More Specific Class(target class=w375, reference=w376) -> (specific class reference=w374:refnum<vi>)  [unwired: 1 in, 1 out]
          n189 = property class="Clust"(reference=w374) -> ("Controls[]"=w373:refnum<vi>[])  [unwired: 1 in, 2 out]
          n190 = Index Array(array=w373, index #1=1 ("index"), index #2=2 ("index")) -> (element #1=w371:refnum<vi>, element #2=w366:refnum<vi>)
          n191 = property class="Ctl"(reference=w371) -> ("Value"=w370:variant)  [unwired: 1 in, 2 out]
          n192 = Variant To Data(type=2, Variant=w370) -> (data=w368:i32)  [unwired: 1 in, 1 out]
          n193 = case shown="2" w368 {
            tunnel: w366 -> [_ w378]
            tunnel: w365 -> [_ w377]
            frame 0, Default {
            }
            frame 2 {
              n194 = property class="Ctl"(reference=w378, "Value"=w377) -> ()  [unwired: 1 in, 2 out]
            }
          }
        }
        n195 = call "FileRefFGV.vi"("Action"=enum16{"Set", "Get", "Initial", "Change"}."Change") -> ()  [unwired: 9 in, 2 out]
      }
      frame "CohortQuickState" {
        n196 = property on="Basic Unit" class="Clust (strict)"() -> ("Controls[]"=w384:refnum<vi>[])  [unwired: 2 in, 2 out]
        n197 = Select(t=0, s="SetHiZ", f=0) -> (s? t:f=w390:i32)
        n198 = Select(t=1, s="SetAnode", f=0) -> (s? t:f=w389:i32)
        n199 = Select(t=2, s="SetCathode", f=0) -> (s? t:f=w388:i32)
        n200 = Compound Arithmetic op=ADD(w390, w389, w388) -> (w383:i32)
        n201 = for {
          tunnel: w384 -> [w404] mode=indexing
          tunnel: w383 -> [w400]
          w403 = refnum<vi> refnum  # Cluster
          n202 = To More Specific Class(target class=w403, reference=w404) -> (specific class reference=w402:refnum<vi>)  [unwired: 1 in, 1 out]
          n203 = property class="Clust"(reference=w402) -> ("Controls[]"=w401:refnum<vi>[], "DisabledEnum"=w397:T12)  [unwired: 1 in, 2 out]
          n204 = Index Array(array=w401, index=1) -> (element=w398:refnum<vi>)
          n205 = case shown="\"Enabled\"" w397 {
            tunnel: w398 -> [_ w406]
            tunnel: w400 -> [_ w405]
            frame Default {
            }
            frame "Enabled" {
              n206 = property class="Ctl"(reference=w406, "Value"=w405) -> ()  [unwired: 1 in, 2 out]
            }
          }
        }
        n207 = call "FileRefFGV.vi"("Action"=enum16{"Set", "Get", "Initial", "Change"}."Change") -> ()  [unwired: 9 in, 2 out]
      }
      frame "Initializing" {
        w417 = refnum<k0> refnum
        w420 = u8 1 ("Set Pulse Frequency")
        w412 = 0
        # "Empty global variables"
        # "Update system status"
        # "Building a empty cohort for initializing"
        n208 = global write "InputPadRef.vi" "NumControl"(w417) -> ()
        n209 = global write "RefWorkingFile.vi" "Working File Refnum"(w417) -> ()
        n210 = call "ReadTime.vi"("Input"="Initializing...", "Status in"=w415) -> ("Status out"=w414:refnum<vi>)  [unwired: 7 in]
        n211 = property on="Select a Cohort to Edit" class="Ring (strict)"("StringsAndValues[]"=T13 [{"String"="Cohort 0", "Value"=0}] ("Strings And Values []"), "Value"=w412) -> ()  [unwired: 2 in, 2 out]
        n212 = control-ref of="Pool"() -> (w407:refnum<vi>)
        n213 = call "SEQPoolFGV.vi"("Action"=T10."Initial") -> ("SEQ out"=w408:refnum<class "Sequence.lvclass">[])  [unwired: 10 in]
        n214 = call "FileRefFGV.vi"("Action"=enum16{"Set", "Get", "Initial", "Change"}."Initial") -> ()  [unwired: 9 in, 2 out]
        n215 = call "CorIndexFGV.vi"("Action"=enum16{"Set", "Get", "Del"}."Set", "Cohort Index"=w412) -> ()  [unwired: 9 in, 1 out]
        n216 = call "SEQPool.vi"("Pool in"=w407, "SEQ in"=w408) -> ()  [unwired: 8 in, 1 out]
        n217 = Initialize Array(-1, 16 ("dimension size")) -> (w421:i32[])
        n218 = call "CohortSet.vi"("Set COR Tag"="This is a cohort", "Set Electrodes"=w421, "Set Pulse Width"=w420, "Set Pulse Frequency"=w420) -> ("Cohort out"=w419:refnum<class "Cohort.lvclass">)  [unwired: 6 in, 1 out]
        n219 = Build Array(w419) -> (w418:refnum<class "Cohort.lvclass">[])
      }
      frame "PoolUpdate" {
        n220 = case shown="False" "Pool Remove" {
          tunnel: [w443 errorcluster {"status"=FALSE, "code"=0, "source"=""} ("error out")] -> w431
          tunnel: w427 -> [_ w451]
          tunnel: [w432 w451] -> w426
          frame False {
            # "To open a SEQ file and add it into the POOL"
            n221 = call "SEQPoolFGV.vi"("Action"=enum16{"Add", "New", "Del", "Update", "Get"}."Get") -> ("SEQ out"=w441:refnum<class "Sequence.lvclass">[])  [unwired: 10 in]
            n222 = Open/Create/Replace File(prompt="Open a Sequence File" ("prompt (Open existing file)"), operation (0:open)=T9."open", access (0:read/write)=enum16{"read/write", "read-only", "write-only"}."read-only") -> (refnum out=w450:refnum<file>, error out=w449:errorcluster)  [unwired: 3 in, 1 out]
            n223 = Array Size(array=w441) -> (size(s)=w440:i32)
            n224 = Equal To 0?(x=w440) -> (x = 0?=w439:bool)
            n225 = call "SeqnRead.vi"("error in (no error)"=w449, "File in Refnum"=w450) -> ("error out"=w444:errorcluster, "SEQ out"=w433:refnum<class "Sequence.lvclass">, "File out Refnum"=w445:refnum<file>)  [unwired: 6 in, 1 out]
            n226 = Select(t=enum16{"Add", "New", "Del", "Update", "Get"}."New" ("Action"), s=w439, f=enum16{"Add", "New", "Del", "Update", "Get"}."Add" ("Action")) -> (s? t:f=w436:enum16{"Add", "New", "Del", "Update", "Get"})
            n227 = call "SEQPoolFGV.vi"("Action"=w436, "SEQ in"=w433) -> ("SEQ out"=w435:refnum<class "Sequence.lvclass">[])  [unwired: 9 in]
            n228 = Close File(refnum=w445, error in=w444) -> (error out=w443:errorcluster)  [unwired: 1 out]
            n229 = control-ref of="Pool"() -> (w434:refnum<vi>)
            n230 = call-dynamic "SeqnGet.vi"("Sequence in"=w433) -> ("Cohorts"=w432:refnum<class "Cohort.lvclass">[])  [unwired: 8 in, 2 out]
            n231 = call "SEQPool.vi"("Pool in"=w434, "SEQ in"=w435) -> ()  [unwired: 8 in, 1 out]
          }
          frame True {
            # "Delete a Sequence from Pool"
            n232 = control-ref of="Pool"() -> (w454:refnum<vi>)
            n233 = property class="Clust (strict)"(reference=w454) -> ("Controls[]"=w453:refnum<vi>[])  [unwired: 1 in, 2 out]
            n234 = flat-sequence {
              tunnel: w452 -> [w457]
              frame #0 {
                n235 = Reverse 1D Array(array=w457) -> (reversed array=w456:dbl[])
                n236 = for {
                  tunnel: w456 -> [w458] mode=indexing
                  n237 = call "SEQPoolFGV.vi"("Action"=enum16{"Add", "New", "Del", "Update"}."Del", "Index"=w458) -> ()  [unwired: 9 in, 1 out]
                }
              }
              frame #1 {
                n238 = control-ref of="Pool"() -> (w461:refnum<vi>)
                n239 = call "SEQPoolFGV.vi"("Action"=T10."Get") -> ("SEQ out"=w460:refnum<class "Sequence.lvclass">[])  [unwired: 10 in]
                n240 = call "SEQPool.vi"("Pool in"=w461, "SEQ in"=w460) -> ()  [unwired: 8 in, 1 out]
              }
            }
            n241 = for {
              tunnel: w453 -> [w473] mode=indexing
              tunnel: [w464] -> w452 mode=indexing
              i -> [w465]
              w470 = u8 0 ("R")
              w472 = refnum<vi> refnum  # Cluster
              n242 = To More Specific Class(target class=w472, reference=w473) -> (specific class reference=w471:refnum<vi>)  [unwired: 1 in, 1 out]
              n243 = property class="Clust"(reference=w471) -> ("Color"=w468:u32)  [unwired: 1 in, 2 out]
              n244 = call <vilib>:"RGB to Color.vi"("B"=u8 196, "G"=w470, "R"=w470) -> ("Color"=w467:u32)
              n245 = Equal?(x=w468, y=w467) -> (x = y?=w466:bool)
              n246 = Select(t=w465, s=w466, f=nan) -> (s? t:f=w464:dbl)
            }
          }
        }
      }
    }
    "error out" <- w5
    n247 = Equal?(x=w11, y=Status."Stop") -> (x = y?=w13:bool)
  }
